vi "Configure Units.vi"(0 "VISA resource name":refnum<visa-resource-name>, 5 "Measurement Type (0: Vacuum)":u16(ring) items=["Vacuum ", "Pressure"], 7 "Pressure Units (0: PSI)":u16(ring) items=["PSI", "BAR", "KPA"], 9 "Vacuum Units (1: inH20)":u16(ring)=1 items=["KPA", "inH2O", "inHg", "mmHg", "TORR"], 11 "error in (no error)":errorcluster) -> (4 "VISA resource name out":refnum<visa-resource-name>, 15 "error out":errorcluster)   [LabVIEW 2020, in "EFD Ultimus V.lvlib"]
doc: "Sets the units the dispenser is using to display pressure and vacuum. Measurement type, selects which unit to change, either pressure or vacuum."
uses:
  EFD Ultimus V.lvlib
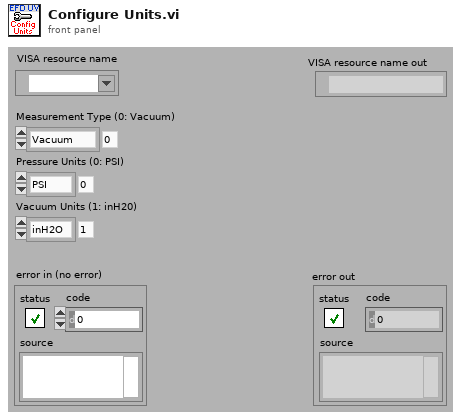
[diagram p1: front panel]
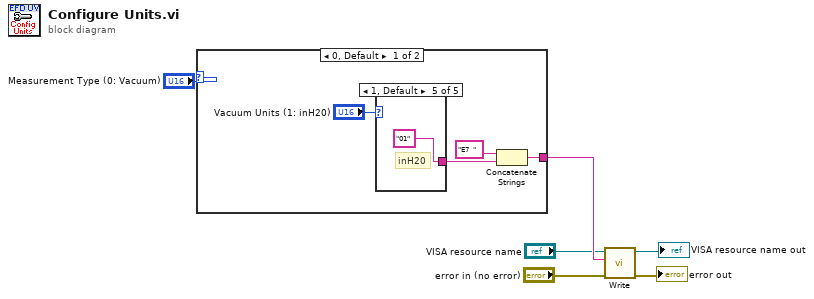
[diagram p0: block diagram]
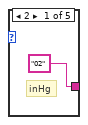
[diagram p2: hidden frame]
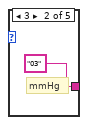
[diagram p3: hidden frame]
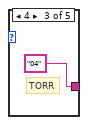
[diagram p4: hidden frame]
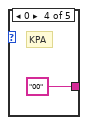
[diagram p5: hidden frame]
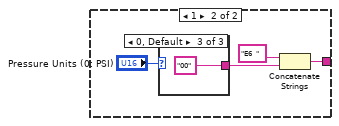
[diagram p6: hidden frame]
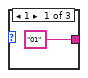
[diagram p7: hidden frame]
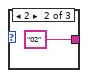
[diagram p8: hidden frame]
diagram:
  n1 = case shown="0, Default" "Measurement Type (0: Vacuum)" {
    tunnel: [w8 w17] -> w6
    frame 0, Default {
      n2 = case shown="1, Default" "Vacuum Units (1: inH20)" {
        tunnel: ["02" ("string") "03" ("string") "04" ("string") "00" ("string") "01" ("string")] -> w9
        frame 2 {
          # "inHg"
        }
        frame 3 {
          # "mmHg"
        }
        frame 4 {
          # "TORR"
        }
        frame 0 {
          # "KPA"
        }
        frame 1, Default {
          # "inH20"
        }
      }
      n3 = Concatenate Strings("E7  " ("string"), w9) -> (w8:string)
    }
    frame 1 {
      n4 = case shown="0, Default" "Pressure Units (0: PSI)" {
        tunnel: ["01" ("string") "02" ("string") "00" ("string")] -> w19
        frame 1 {
        }
        frame 2 {
        }
        frame 0, Default {
        }
      }
      n5 = Concatenate Strings("E6  " ("string"), w19) -> (w17:string)
    }
  }
  n6 = call "Write.vi"("error in (no error)"="error in (no error)", "Command To Write"=w6, "VISA resource name"="VISA resource name") -> ("error out"=→"error out":errorcluster, "VISA resource name out"=→"VISA resource name out":refnum<visa-resource-name>)  [unwired: 7 out]
